vi "Get Repository Base DIR.vi"(8 "error in (no error)":errorcluster, 10 "relative path":string) -> (0 "error out":errorcluster, 2 "repo DIR":string)   [LabVIEW 2020, in "TALOS.lvlib" / "Kasli Wrapper 2.0.lvlib" / "Kasli Wrapper 2.0.lvclass"]
uses:
  Kasli Wrapper 2.0.lvclass
  Kasli Wrapper 2.0.lvclass/Kasli Wrapper 2.0.ctl
  Kasli Wrapper 2.0.lvlib
  Kasli/Kasli.lvclass
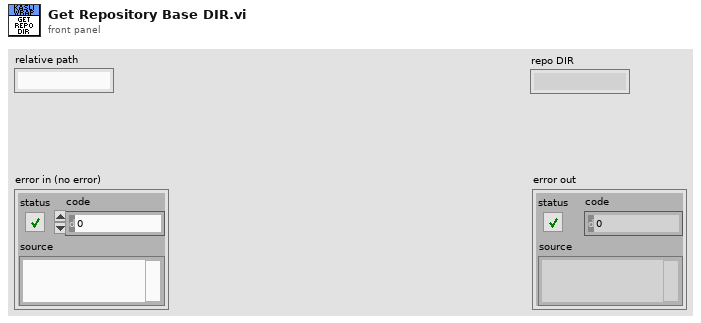
[diagram p1: front panel]
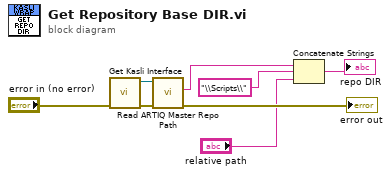
[diagram p0: block diagram]
diagram:
  n1 = call "Get Kasli Interface.vi"("error in"="error in (no error)") -> ("error out"=w2:errorcluster, "Kasli Interface"=w3:refnum<class "Kasli.lvclass">)  [unwired: 9 in]
  n2 = call-dynamic "Read ARTIQ Master Repo Path.vi"("error in (no error)"=w2, "Kasli in"=w3) -> ("error out"=→"error out":errorcluster, "ARTIQ Master Repo Path"=w1:string)  [unwired: 7 in, 1 out]
  n3 = Concatenate Strings(w1, "\\Scripts\\", "relative path") -> (→"repo DIR":string)
